vi "5-1ManupuleArrays.vi"() -> ()   [LabVIEW 2024]
uses:
  <vilib>/measure/NI_MABase.lvlib
panel:
  in  "Stop Button":bool
  in  "Tab Control 2":T1(tab)
  out "Concatenated Data":dbl[](graph)
  out "Concatenated Data Array":dbl[](array[numeric])
  out "Waveform Chart":dbl[](graph)
  out "Waveform Graph":dbl[](graph)
  out "Add":dbl[](graph)
  in  "Boolean":bool
  in  "Select Channel":u16(ring) items=["Channel 0", "Channel 1"]
  out "Single Channel of Data":dbl[](graph)
  out "Size of Array":i32
  out "Concatenated Data Array 2":dbl[](array[numeric])
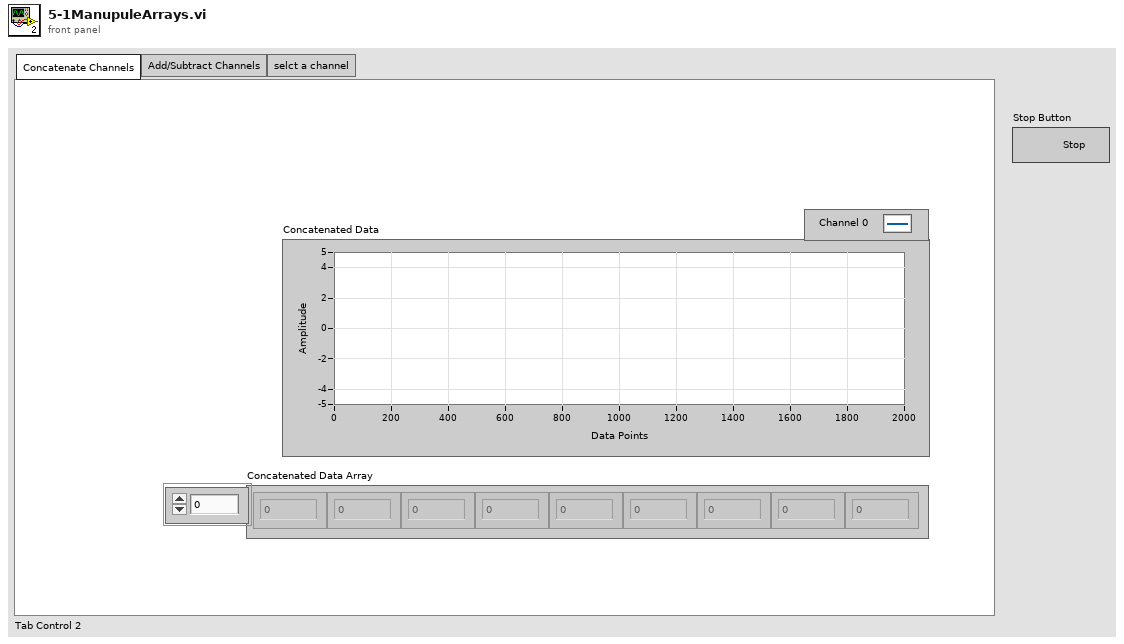
[diagram p1: front panel]
types:
  T1 = enum32{"Concatenate Channels", "Add/Subtract Channels", "selct a channel"}
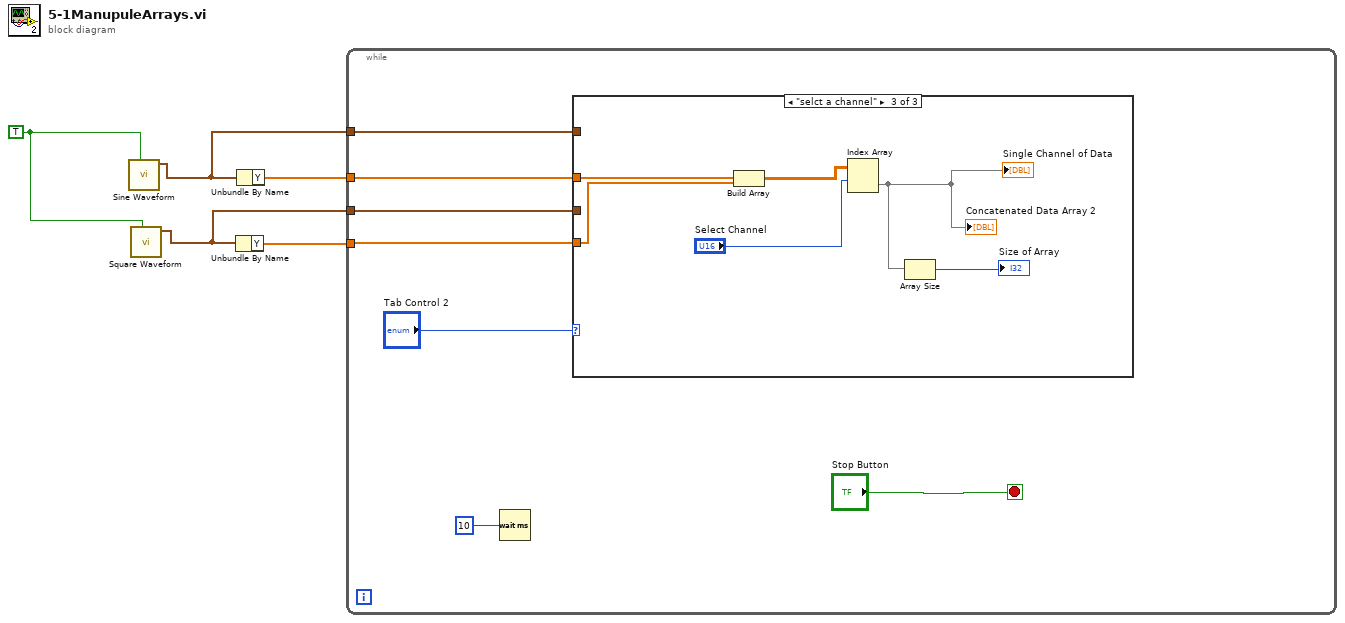
[diagram p0: block diagram]
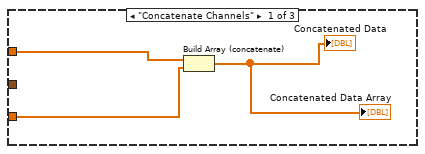
[diagram p2: hidden frame]
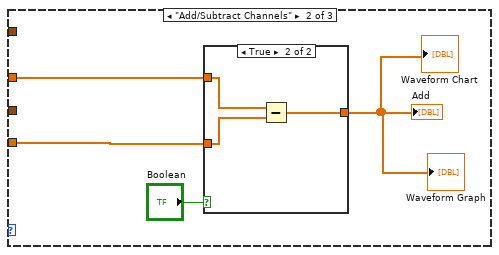
[diagram p3: hidden frame]
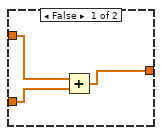
[diagram p4: hidden frame]
diagram:
  w1 = TRUE
  n1 = call <vilib>:"Sine Waveform.vi"("reset signal"=w1) -> ("signal out"=w4:waveform(dbl))  [unwired: 9 in, 1 out]
  n2 = call <vilib>:"Square Waveform.vi"("reset signal"=w1) -> ("signal out"=w2:waveform(dbl))  [unwired: 9 in, 1 out]
  n3 = Unbundle By Name(w2) -> ("Y"=w3:dbl[])
  n4 = Unbundle By Name(w4) -> ("Y"=w5:dbl[])
  n5 = while {
    tunnel: w5 -> [w8]
    tunnel: w4 -> [w9]
    tunnel: w3 -> [w6]
    tunnel: w2 -> [w7]
    stop <- "Stop Button" stop-if-true
    n6 = Wait (ms)(milliseconds to wait=u32 10) -> ()  [unwired: 1 out]
    n7 = case shown="\"selct a channel\"" "Tab Control 2" {
      tunnel: w9 -> [_ _ _]
      tunnel: w8 -> [w15 w18 w31]
      tunnel: w7 -> [_ _ _]
      tunnel: w6 -> [w14 w17 w30]
      frame "Concatenate Channels" {
        n8 = Build Array (concatenate) "Build Array"(w15, w14) -> (→"Concatenated Data" →"Concatenated Data Array":dbl[])
      }
      frame "Add/Subtract Channels" {
        n9 = case shown="True" "Boolean" {
          tunnel: w18 -> [w21 w25]
          tunnel: w17 -> [w22 w24]
          tunnel: [w20 w23] -> w16
          frame False {
            n10 = Add(x=w21, y=w22) -> (x+y=w20:dbl[])
          }
          frame True {
            n11 = Subtract(x=w25, y=w24) -> (x-y=w23:dbl[])
          }
        }
        "Add" <- w16
        "Waveform Graph" <- w16
        "Waveform Chart" <- w16
      }
      frame "selct a channel" {
        n12 = Build Array(w31, w30) -> (w29:dbl[][])
        n13 = Index Array(array=w29, index (row)="Select Channel") -> (element=w27:dbl[])  [unwired: 1 in]
        "Single Channel of Data" <- w27
        "Concatenated Data Array 2" <- w27
        n14 = Array Size(array=w27) -> (size(s)=→"Size of Array":i32)
      }
    }
  }
